vi "Get BC.vi"(8 "error in (no error)":errorcluster, 10 "Domain":refnum<class "NI_Domain.lvclass">, 11 "BC in":refnum<class "NI_BC.lvclass">) -> (0 "error out":errorcluster, 2 "BC":variant, 3 "BC out":refnum<class "NI_BC.lvclass">)   [LabVIEW 2020, in "NI_PDE.lvlib" / "NI_BC.lvclass"]
uses:
  <vilib>/gmath/pde.llb/BCClass/NI_BC.lvclass
  <vilib>/gmath/pde.llb/DomainClass/NI_Domain.lvclass
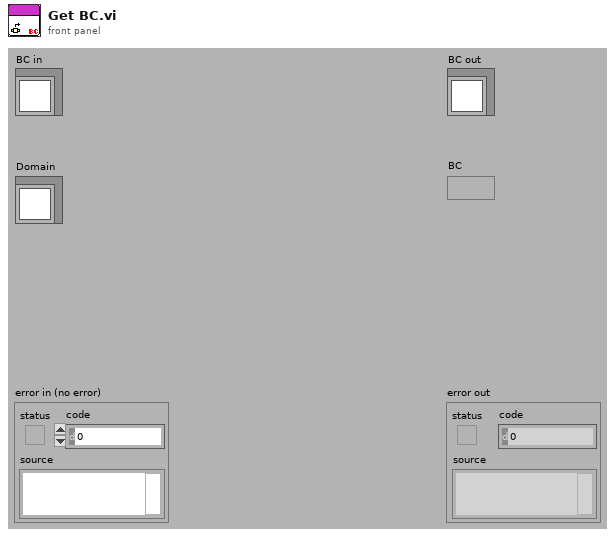
[diagram p1: front panel]
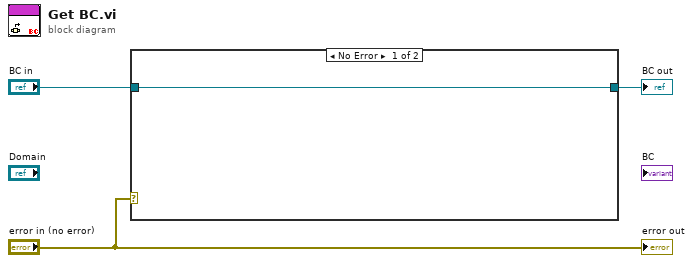
[diagram p0: block diagram]
diagram:
  n1 = case shown="No Error" "error in (no error)" {
    tunnel: "BC in" -> [w4 w5]
    tunnel: [w4 w5] -> w2
    frame No Error {
    }
    frame Error {
    }
  }
  "BC out" <- w2
  "error out" <- "error in (no error)"
